vi "Release Queue.vi"(8 "error in (no error)":errorcluster, 10 "TAS_Message.lvclass":refnum<class "TAS_Message.lvclass">, 11 "Queue Name":string) -> (0 "error out":errorcluster, 2 "remaining elements":refnum<class "TAS_Message.lvclass">[](array[class]), 3 "queue name":string)   [LabVIEW 2012, in "TAS_Message.lvclass"]
uses:
  TAS_Message.lvclass
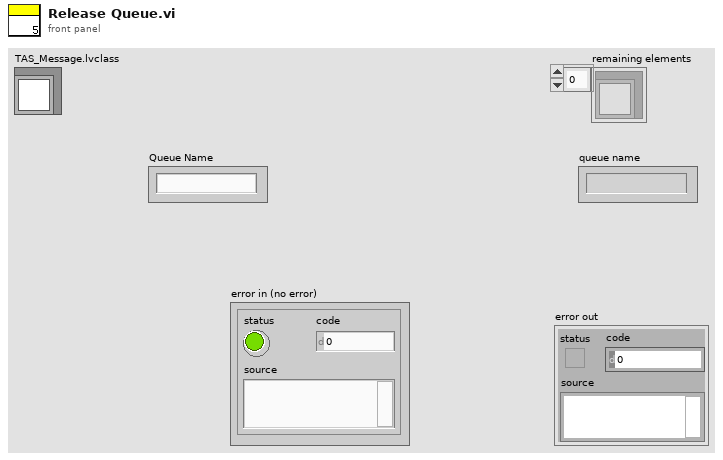
[diagram p1: front panel]
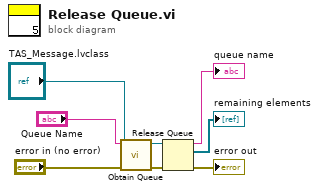
[diagram p0: block diagram]
diagram:
  n1 = call-dynamic "Obtain Queue.vi"("error in (no error)"="error in (no error)", "TAS_Message.lvclass"="TAS_Message.lvclass", "Queue Name"="Queue Name") -> ("error out"=w5:errorcluster, "queue out"=w6:refnum<queue>)  [unwired: 7 in]
  n2 = Release Queue(queue=w6, error in (no error)=w5) -> (queue name=→"queue name":string, remaining elements=→"remaining elements":refnum<class "TAS_Message.lvclass">[], error out=→"error out":errorcluster)  [unwired: 1 in]
